vi "Find Enemy.vi"(4 "Y":i32, 6 "X":i32, 9 "attack array":bool[][](array[boolean]), 10 "View":i32[](array[numeric]), 11 "Team Index":i32) -> (2 "Direction":T1, 3 "Found Enemy?":bool)   [LabVIEW 2015, in "Uno.lvclass"]
uses:
  Uno.lvclass
  Type Defs/Direction Enum.ctl
  Type Defs/SB Type Defs.lvlib
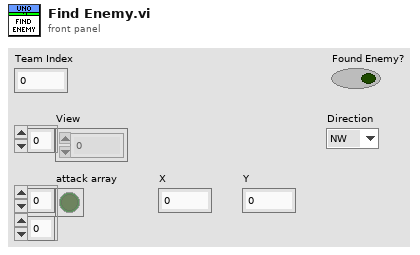
[diagram p1: front panel]
types:
  T1 = typedef "SB Type Defs.lvlib/Direction Enum.ctl" = enum16{"NW", "N", "NE", "E", "SE", "S", "SW", "W"}
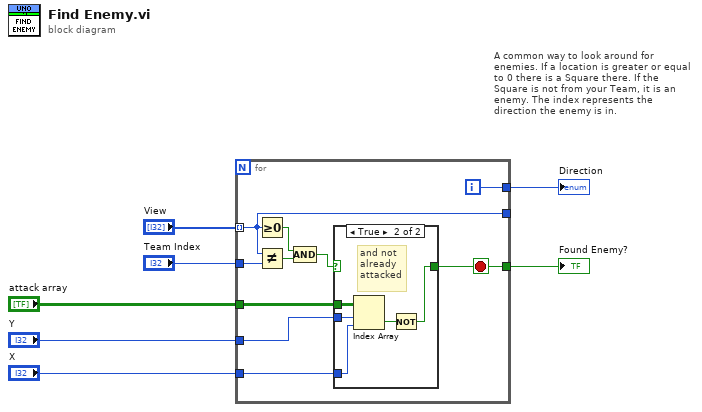
[diagram p0: block diagram]
diagram:
  # "A common way to look around for enemies. If a location is greater or equal to 0 there is a Square there. If the Square is not from your Team, it is an enemy. The index represents the direction the enemy is in."
  n1 = for {
    tunnel: "View" -> [w13] mode=indexing
    tunnel: "Team Index" -> [w16]
    tunnel: [w14] -> w7
    tunnel: [w11] -> w6
    tunnel: [w13] -> _
    tunnel: "attack array" -> [w10]
    tunnel: "Y" -> [w9]
    tunnel: "X" -> [w8]
    i -> [w14]
    stop <- w11 stop-if-true
    n2 = Greater Or Equal To 0?(x=w13) -> (x >= 0?=w17:bool)
    n3 = Not Equal?(x=w13, y=w16) -> (x != y?=w15:bool)
    n4 = Compound Arithmetic op=AND(w17, w15) -> (w12:bool)
    n5 = case shown="True" w12 {
      selector: w12 -> [w18 _]
      tunnel: [w18 w19] -> w11
      tunnel: w10 -> [_ w23]
      tunnel: w9 -> [_ w22]
      tunnel: w8 -> [_ w21]
      frame False {
      }
      frame True {
        # "and not\nalready\nattacked"
        n6 = Index Array(array=w23, index (row)=w22, index (col)=w21) -> (element=w20:bool)
        n7 = Not(x=w20) -> (.not. x?=w19:bool)
      }
    }
  }
  "Direction" <- w7
  "Found Enemy?" <- w6
